vi "Get Create TDMS Path.vi"() -> (3 "tdms file path":path)   [LabVIEW 2022 SP3, in "DAQ.lvclass"]
doc: "Developed by Kevin Thompson\nkevin@thompsonengineering.net\n\nCopyright 2018-2020\nThompson Engineering, LLC"
uses:
  DAQ.lvclass
  DAQ.lvclass/DAQ.ctl
  DAQ_Common/DataTypes/TD GetSet ActionSelect--enum.ctl
panel:
  out "error out":errorcluster
  in  "error in (no error)":errorcluster
  out "relative date folder":string
  out "time":string
  out "Day path":path
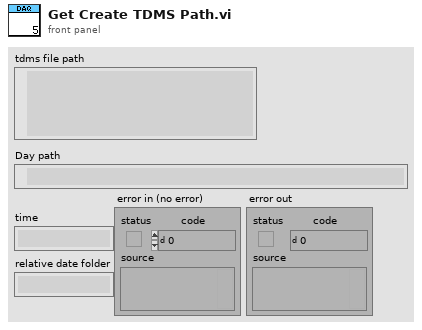
[diagram p1: front panel]
types:
  T1 = typedef "TD GetSet ActionSelect--enum.ctl" = enum16{"Init", "Get", "Set"}
  T2 = typedef "TD Pathnames--cluster.ctl" = cluster{"RunTimeSys?":bool, "AppFolder":path, "ExecutablePath":path, "ConfigFolder":path, "DataLogFolder":path, "SystemLogFolder":path, "SeqFolder":path, "MainStartupPathname":path, "MainUIPathname":path, "SystemEventsFile":path, "SeqEventsFile":path, "Config SettingsFile":path, "DAQ IOConfigFile":path, "SystemSimulation":bool}
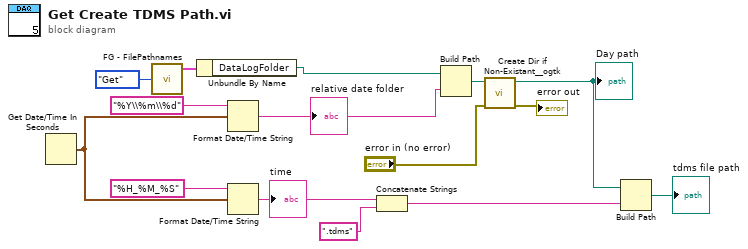
[diagram p0: block diagram]
diagram:
  n1 = Get Date/Time In Seconds() -> (seconds since 1Jan1904=w11:timestamp)
  n2 = call "FG - FilePathnames.vi"("action (Get)"=TD_GetSet_ActionSelect--enum."Get") -> ("FilePaths out"=w15:T2)  [unwired: 3 in, 1 out]
  n3 = Unbundle By Name(w15) -> ("DataLogFolder"=w9:path)
  n4 = Format Date/Time String(time format string (%c)="%Y\\%m\\%d", seconds (now)=w11) -> (date/time string=w10:string)  [unwired: 1 in]
  "relative date folder" <- w10
  n5 = Format Date/Time String(time format string (%c)="%H_%M_%S", seconds (now)=w11) -> (date/time string=w8:string)  [unwired: 1 in]
  "time" <- w8
  n6 = Concatenate Strings(w8, ".tdms" ("string")) -> (w6:string)
  n7 = Build Path(base path=w9, name or relative path=w10) -> (appended path=w4:path)
  n8 = call <userlib>:"Create Dir if Non-Existant__ogtk.vi"("error in (no error)"="error in (no error)", "Directory Path"=w4) -> ("error out"=→"error out":errorcluster, "dup Directory Path"=w3:path)  [unwired: 7 in, 1 out]
  "Day path" <- w3
  n9 = Build Path(base path=w3, name or relative path=w6) -> (appended path=→"tdms file path":path)
